vi "Anchor Object Array to Cluster Array.vi"(8 "error in (no error)":errorcluster, 11 "AnchorArray In":refnum<class "Anchor.lvclass">[](array[class])) -> (0 "error out":errorcluster, 3 "AnchorArray Out":T1(array[cluster]))   [LabVIEW 2014]
uses:
  Anchor.lvclass
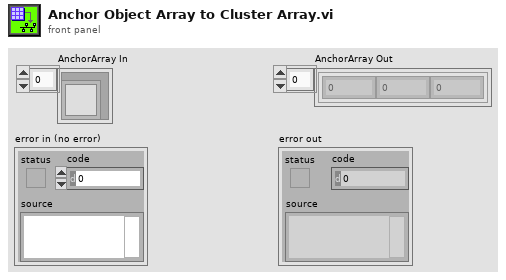
[diagram p1: front panel]
types:
  T1 = cluster{"AnchorID":dbl, "AnchorX":dbl, "AnchorY":dbl}[]
  T2 = cluster{"AnchorID":dbl, "AnchorX":dbl, "AnchorY":dbl}
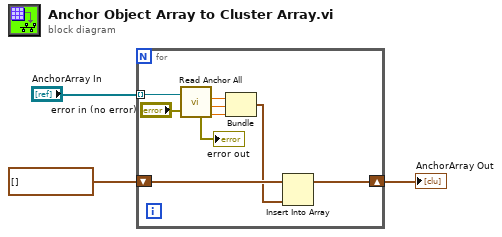
[diagram p0: block diagram]
diagram:
  n1 = for {
    tunnel: "AnchorArray In" -> [w12] mode=indexing
    shift-right: [w6] -> w1
    shift-left: T1 [] ("AnchorArray Out 2") -> [w5]
    n2 = call-dynamic "Read Anchor All.vi"("error in (no error)"="error in (no error)", "Anchor in"=w12) -> ("AnchorY"=w7:dbl, "AnchorX"=w8:dbl, "AnchorID"=w9:dbl, "error out"=→"error out":errorcluster)  [unwired: 1 out]
    n3 = Bundle("AnchorID"=w9, "AnchorX"=w8, "AnchorY"=w7) -> (w4:T2)  [unwired: 1 in]
    n4 = Insert Into Array(array=w5, new element=w4) -> (w6:T1)  [unwired: 1 in]
  }
  "AnchorArray Out" <- w1
